vi "LCSS classification loop.vi"() -> ()   [LabVIEW 2013]
panel:
  in  "Left":string[](array[string])
  in  "ALL":string[](array[string])
  out "output array":i32[][](array[numeric])
  in  "All":i32[](array[numeric])
  in  "Right":i32[](array[numeric])
  in  "Left":i32[](array[numeric])
  out "Cluster element count 2":i32[](array[numeric])
  in  "CJ ALL 5":string[](array[string])
  in  "CJ right 3":string[](array[string])
  in  "CJ right 5":string[](array[string])
  in  "CJ left 3":string[](array[string])
  in  "CJ left 5":string[](array[string])
  in  "CJ ALL 3":string[](array[string])
  in  "Array 2":string[](array[string])
  out "Array":i32[](array[numeric])
  out "disabled index (col)":i32
  out "appended array 3":string[][](array[string])
  in  "cluster centers":string[][](array[string])=[["1 0 1", "-1 0 -1", "2 0 4 0 2"], ["2 0 2", "-3 0 -3", "1 0 3 0 1"], ["3 0 3", "-4 0 -4", "1 0 4 0 1"], ["4 0 4", "-2 0 -2", "2 0 3 0 2"]]
  in  "Patterns in":string[](array[string])=["0 4 0", "4 0 4", "0 4 0", "4 0 4", "0 4 0", "4 0 4", "0 4 0", "4 0 -2", "0 -2 3", "-2 3 0", "3 0 3", "0 3 0", "3 0 4", "0 4 0", "-2 0 1", "0 1 0", "1 0 -4", "0 -4 4", "-2 2 0", "2 0 -1", "0 -1 -4", "-1 -4 1", "-4 1 0", "1 0 3", "0 3 0", "-1 0 -1", "0 -1 2", "0 -1 1", "-1 1 0", "1 0 4", "0 4 0", "4 0 3", "0 3 -2", "3 -2 0", "-2 0 -2", "0 -2 3", "-2 3 -2", "3 -2 0", "-2 0 4", "0 4 0", "4 0 -2", "0 -2 2", "2 -1 0", "-1 0 4", "0 4 0", "4 0 2", "0 2 0", "2 0 -2", "0 -2 0", "1 -1 0", "-1 0 3", "0 3 0", "3 0 -4", "0 -4 4", "-4 4 -4", "4 -4 0", "2 -1 0", "-1 0 3", "0 3 -2", "3 -2 0", "-2 0 -3", "0 -3 0", "-3 0 3", "0 3 0", "3 0 -3", "0 -3 0", "0 4 0", "4 0 4", "0 4 -4", "4 -4 1", "-4 1 -1", "1 -1 0", "-1 0 -3", "0 -3 0", "-3 0 1", "0 1 -4", "1 -4 1", "-4 1 0", "1 0 4", "0 4 0", "4 0 -4", "0 -4 0", "-4 0 -4", "0 -4 4", "-4 4 -4", "4 -4 1", "0 -4 1", "-4 1 0", "1 0 -4", "0 -4 4", "0 4 0", "4 0 -2", "0 -2 2", "-2 2 -2", "2 -2 2", "-2 2 -2", "2 -2 2", "-2 2 -1", "2 -1 0", "-1 0 4", "0 4 0", "4 0 2", "0 2 0", "2 0 4", "0 4 0", "4 0 2", "0 2 -2", "2 -2 0", "-2 0 4", "1 0 -1", "0 -1 0", "-1 0 -1", "0 -1 0", "-1 0 1", "0 1 -1", "-2 2 -2", "2 -2 3", "1 0 -1", "0 -1 0", "-1 0 -1", "0 -1 2", "-1 2 0", "2 0 2", "0 2 -2", "2 -2 0", "-2 0 -4", "0 -4 0", "-2 2 0", "2 0 3", "0 3 -2", "3 -2 2", "1 -1 0", "-1 0 3", "0 4 0", "-2 0 1", "0 1 -4", "1 -4 0", "-4 0 -3", "0 -3 0", "1 0 -1", "0 -1 2", "-1 2 -1", "2 -1 1", "-1 1 -4", "-2 0 -1", "0 -1 1", "0 3 0", "3 0 3", "0 3 0", "3 0 3", "0 3 -2", "-4 0 -4", "0 -4 4", "0 4 0", "4 0 -4", "0 -4 0", "-4 0 -4", "-2 2 0", "2 0 4", "0 4 -4", "4 -4 0", "-4 0 2", "0 2 -2"]
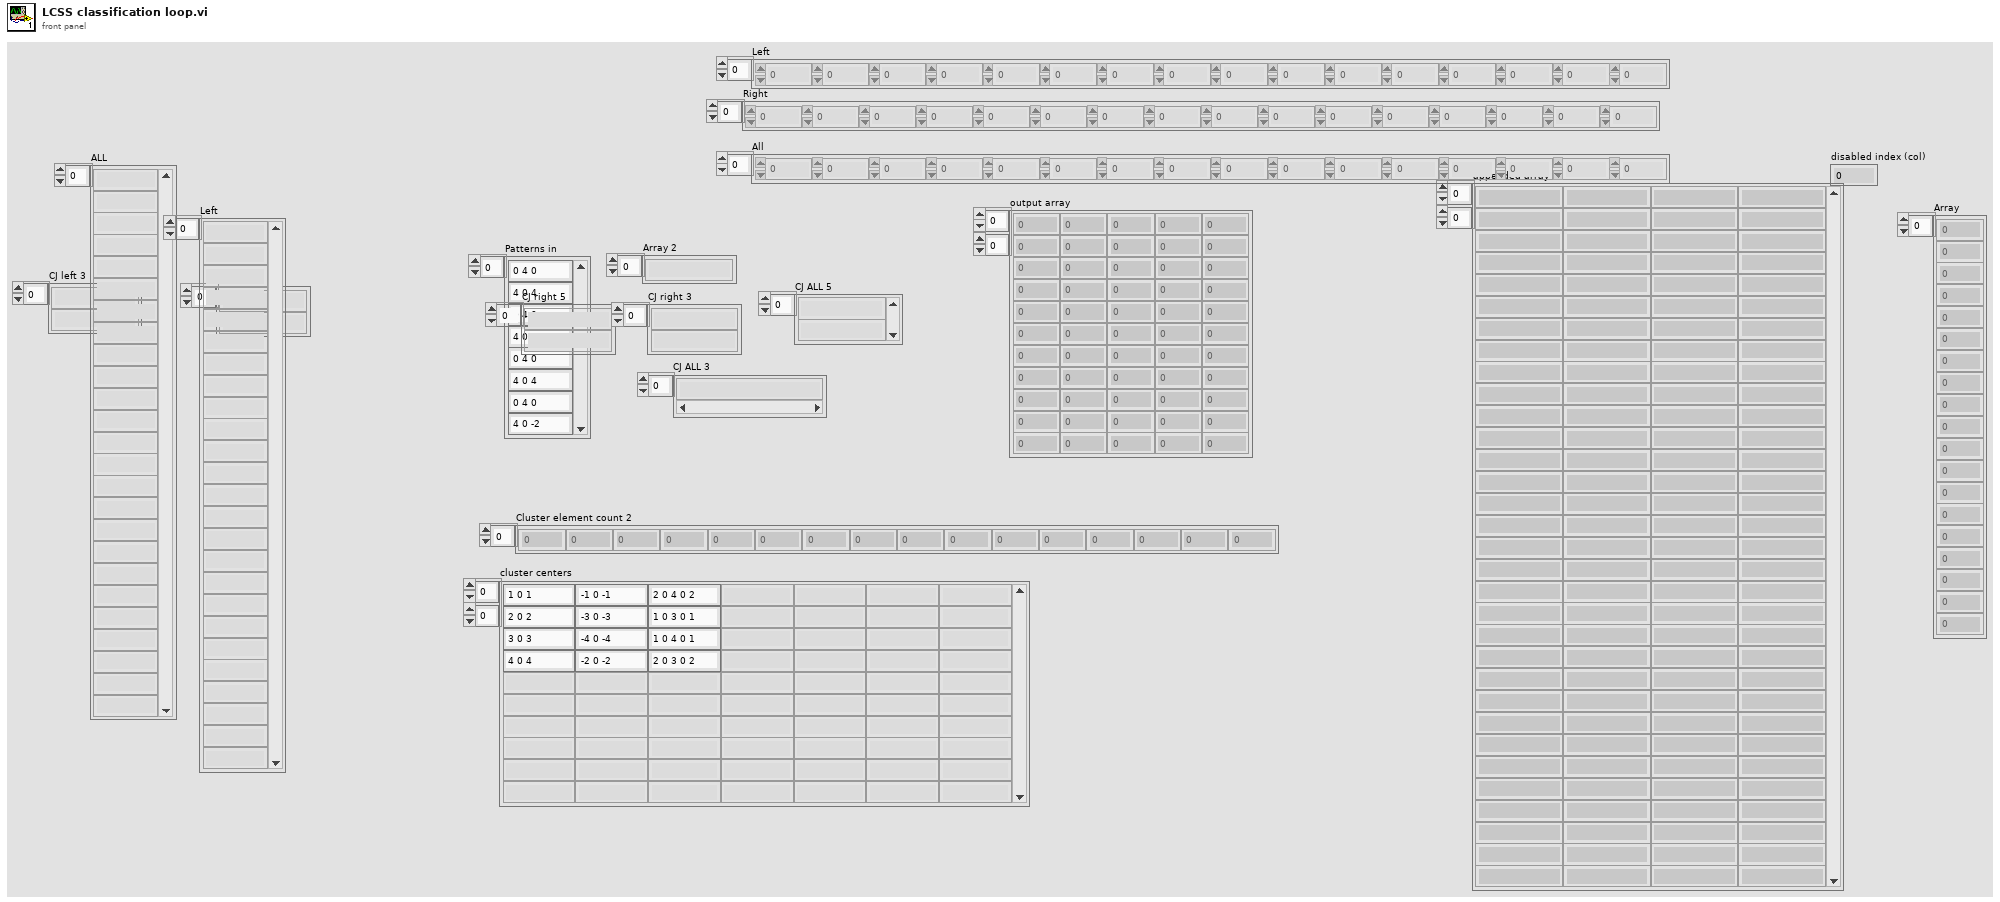
[diagram p1: front panel]
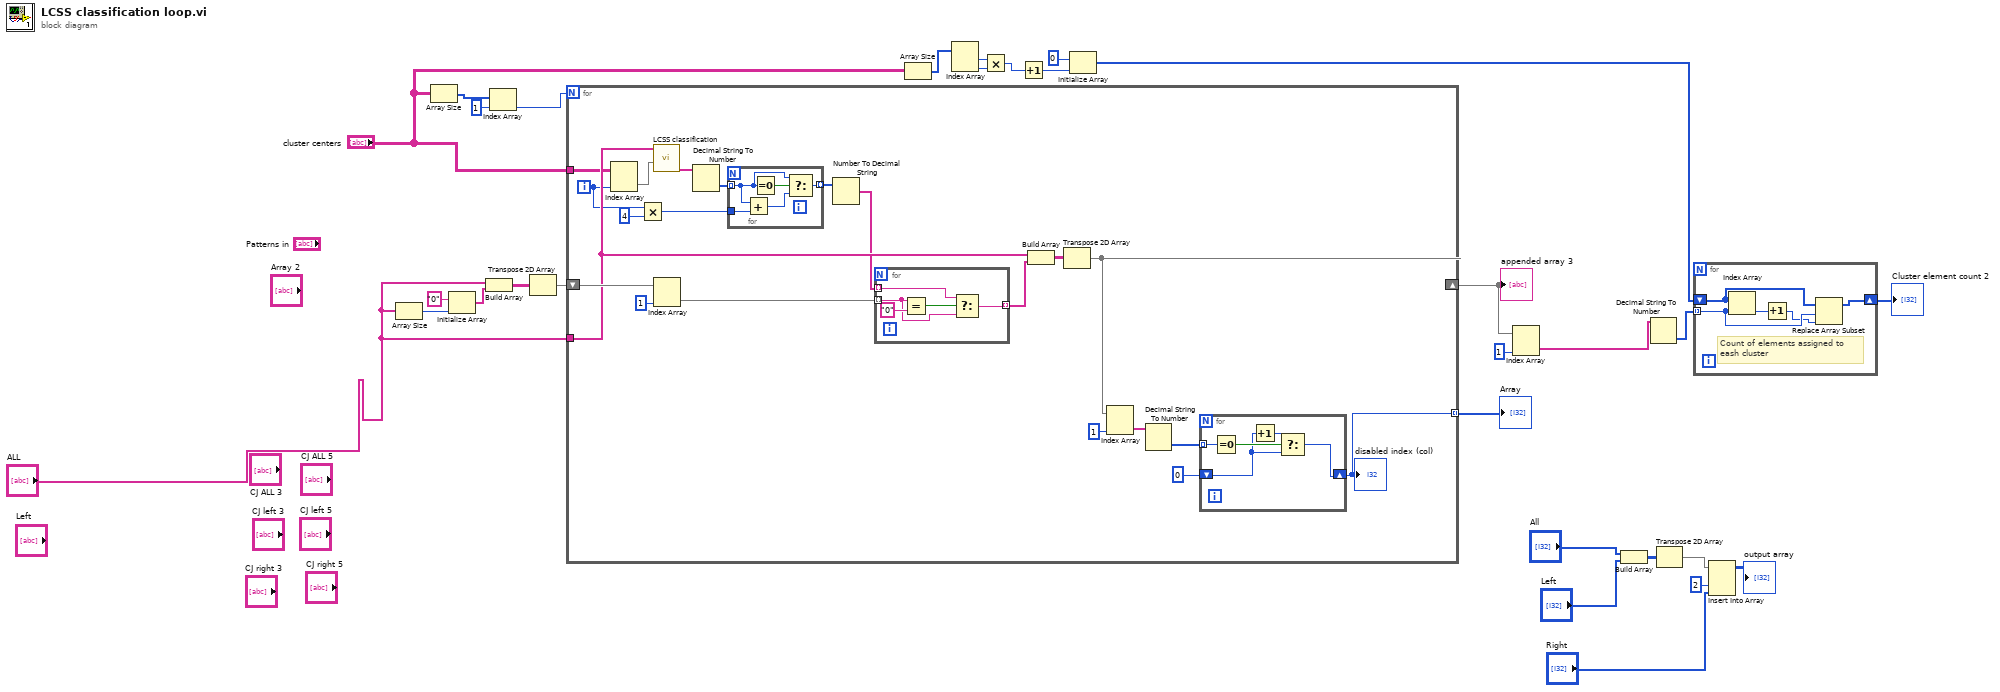
[diagram p0: block diagram]
diagram:
  n1 = Array Size(array="ALL") -> (size(s)=w27:i32)
  n2 = Array Size(array="cluster centers") -> (size(s)=w25:i32[])
  n3 = Initialize Array("0" ("spreadsheet string"), w27) -> (w29:string[])
  n4 = Build Array("ALL", w29) -> (w28:string[][])
  n5 = Index Array(array=w25, index=1) -> (element=w22:i32)
  n6 = Transpose 2D Array(2D array=w28) -> (transposed array=w26:string[][])
  n7 = for {
    N: w22 -> [_]
    tunnel: "ALL" -> [w48]
    tunnel: "cluster centers" -> [w45]
    shift-right: [w43] -> w15
    shift-left: w26 -> [w51]
    tunnel: [w38] -> w23 mode=indexing
    i -> [w36]
    n8 = Index Array(array=w45, index (col)=w36) -> (element=w44:string[])  [unwired: 1 in]
    n9 = Multiply(x=w36, y=4) -> (x*y=w34:i32)
    n10 = call "LCSS classification.vi"("cluster centers"=w44, "Patterns in"=w48) -> ("Assigned cluster (0) unassigned"=w32:string[])  [unwired: 7 in, 2 out]
    n11 = Index Array(array=w51, index (col)=1 ("disabled index (col)")) -> (element=w49:string[])  [unwired: 1 in]
    n12 = Decimal String To Number(string=w32) -> (number=w37:i32[])  [unwired: 2 in, 1 out]
    n13 = for {
      tunnel: w37 -> [w53] mode=indexing
      tunnel: w34 -> [w56]
      tunnel: [w52] -> w33 mode=indexing
      n14 = Add(x=w53, y=w56) -> (x+y=w55:i32)
      n15 = Equal To 0?(x=w53) -> (x = 0?=w54:bool)
      n16 = Select(t=w53, s=w54, f=w55) -> (s? t:f=w52:i32)
    }
    n17 = Number To Decimal String(number=w33) -> (decimal integer string=w31:string[])  [unwired: 1 in]
    n18 = for {
      tunnel: w49 -> [w63] mode=indexing
      tunnel: w31 -> [w64] mode=indexing
      tunnel: [w62] -> w47 mode=indexing
      n19 = Equal?(x=w63, y="0") -> (x = y?=w65:bool)
      n20 = Select(t=w64, s=w65, f=w63) -> (s? t:f=w62:string)
    }
    n21 = Build Array(w48, w47) -> (w46:string[][])
    n22 = Transpose 2D Array(2D array=w46) -> (transposed array=w43:string[][])
    n23 = Index Array(array=w43, index (col)=1 ("disabled index (col)")) -> (element=w41:string[])  [unwired: 1 in]
    n24 = Decimal String To Number(string=w41) -> (number=w40:i32[])  [unwired: 2 in, 1 out]
    n25 = for {
      tunnel: w40 -> [w61] mode=indexing
      shift-right: [w58] -> w38
      shift-left: 0 ("disabled index (col)") -> [w57]
      n26 = Equal To 0?(x=w61) -> (x = 0?=w60:bool)
      n27 = Increment(x=w57) -> (x+1=w59:i32)
      n28 = Select(t=w59, s=w60, f=w57) -> (s? t:f=w58:i32)
    }
    "disabled index (col)" <- w38
  }
  "appended array 3" <- w15
  "Array" <- w23
  n29 = Array Size(array="cluster centers") -> (size(s)=w12:i32[])
  n30 = Index Array(array=w12) -> (element #1=w11:i32, element #2=w10:i32)  [unwired: 2 in]
  n31 = Multiply(x=w11, y=w10) -> (x*y=w9:i32)
  n32 = Increment(x=w9) -> (x+1=w19:i32)
  n33 = Initialize Array(0 ("index"), w19) -> (w16:i32[])
  n34 = Index Array(array=w15, index (col)=1 ("disabled index (col)")) -> (element=w13:string[])  [unwired: 1 in]
  n35 = Build Array("All", "Left") -> (w6:i32[][])
  n36 = Decimal String To Number(string=w13) -> (number=w20:i32[])  [unwired: 2 in, 1 out]
  n37 = Transpose 2D Array(2D array=w6) -> (transposed array=w5:i32[][])
  n38 = for {
    tunnel: w20 -> [w69] mode=indexing
    shift-right: [w67] -> w21
    shift-left: w16 -> [w70]
    # "Count of elements assigned to \neash cluster"
    n39 = Index Array(array=w70, index=w69) -> (element=w71:i32)
    n40 = Increment(x=w71) -> (x+1=w68:i32)
    n41 = Replace Array Subset(array=w70, new element=w68, index=w69) -> (w67:i32[])
  }
  "Cluster element count 2" <- w21
  n42 = Insert Into Array(array=w5, index (col)=2 ("disabled index (col)"), new element="Right") -> (→"output array":i32[][])  [unwired: 1 in]
